vi "Main.vi"() -> ()   [LabVIEW 2019]
uses:
  Support/Gamepad.ctl
  Support/Color.ctl
  Support/Control Panel Motors.ctl
panel:
  out "Arm In":bool
  out "Arm Out":bool
  out "Color":T1
  in  "stop":bool
  in  "Gamepad":T2={"A"=FALSE, "B"=FALSE, "X"=FALSE, "Y"=FALSE, "LB"=FALSE, "RB"=FALSE, "Back"=FALSE, "Next"=FALSE, "Left Stick X"=0.0, "Left Stick Y"=0.0, "Right Stick X"=0.0, "Right Stick Y"=0.0, "LT"=1.0, "RT"=1.0, "D-Pad X"=0, "D-Pad Y"=0} {"Left Stick X" scale=-1.0..1.0; "Left Stick Y" scale=1.0..-1.0; "Right Stick X" scale=-1.0..1.0; "Right Stick Y" scale=1.0..-1.0; "D-Pad Y" step=1 scale=1.0..-1.0; "D-Pad X" step=1 scale=-1.0..1.0; "LT" scale=1.0..-1.0; "RT" scale=1.0..-1.0}
  out "Control Panel Motor":dbl(slide) scale=-1.0..1.0
  out "Arm Motor":dbl(slide) scale=-1.0..1.0
  out "Control Panel Full":dbl
  out "Control Panel":dbl(knob) scale=0.0..1.0
  out "Arm":dbl(knob) scale=0.0..1.0
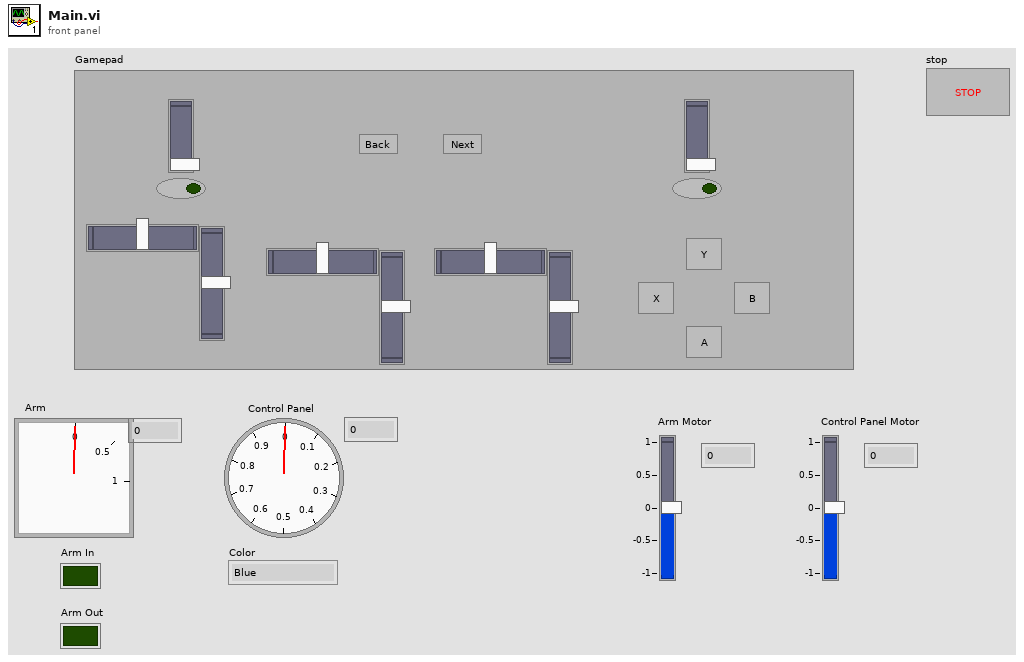
[diagram p1: front panel]
types:
  T1 = typedef "Color.ctl" = enum16{"Blue", "Green", "Red", "Yellow"}
  T2 = typedef "Gamepad.ctl" = cluster{"A":bool, "B":bool, "X":bool, "Y":bool, "LB":bool, "RB":bool, "Back":bool, "Next":bool, "Left Stick X":dbl, "Left Stick Y":dbl, "Right Stick X":dbl, "Right Stick Y":dbl, "LT":dbl, "RT":dbl, "D-Pad X":i32, "D-Pad Y":i32}
  T3 = typedef "Control Panel Motors.ctl" = cluster{"Arm":dbl, "Wheel":dbl}
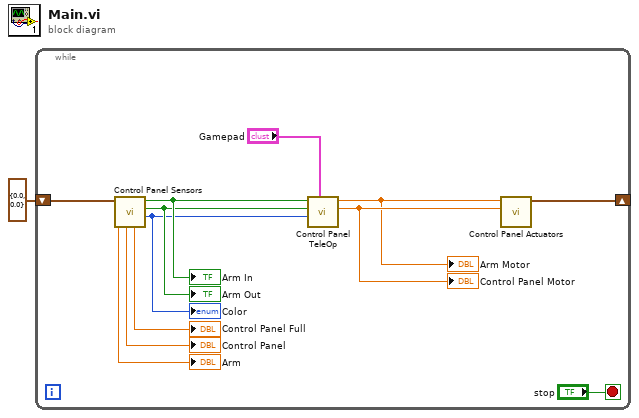
[diagram p0: block diagram]
diagram:
  n1 = while {
    shift-right: [w13] -> _
    shift-left: T3 {"Arm"=0.0, "Wheel"=0.0} ("Color Wheel Motors") -> [w12]
    stop <- "stop" stop-if-true
    n2 = call "Control Panel Sensors.vi"("Control Panel Motors"=w12) -> ("Color"=w9:T1, "Arm Out"=w10:bool, "Arm In"=w11:bool, "Control Panel Full"=→"Control Panel Full":dbl, "Control Panel"=→"Control Panel":dbl, "Arm"=→"Arm":dbl)  [unwired: 5 in]
    "Color" <- w9
    "Arm Out" <- w10
    "Arm In" <- w11
    n3 = call "Control Panel TeleOp.vi"("Gamepad"="Gamepad", "Color"=w9, "Arm Out"=w10, "Arm In"=w11) -> ("Wheel"=w5:dbl, "Arm"=w4:dbl)  [unwired: 6 in]
    "Arm Motor" <- w4
    "Control Panel Motor" <- w5
    n4 = call "Control Panel Actuators.vi"("Wheel"=w5, "Arm"=w4) -> ("Control Panel Motors"=w13:T3)  [unwired: 9 in]
  }
